vi "FPGA_initialize.vi"(2 "error in":errorcluster) -> (0 "error out":errorcluster)   [LabVIEW 2015]
uses:
  <vilib>/FPGAPlugInAG/PCIe-7841R/niLvFpga_Open_PCIe-7841R.vi
  <vilib>/rvi/interface/common/dynamic/niFpgaDynamicAddResources.vi
  <vilib>/FPGAPlugInAG/Dynamic/niLvFpga_Abort_Dynamic.vi
  <vilib>/FPGAPlugInAG/Dynamic/niLvFpga_Reset_Dynamic.vi
  <vilib>/FPGAPlugInAG/Dynamic/niLvFpga_Close_Dynamic.vi
  <vilib>/rvi/interface/nirviOpenFPGA/nirviOpenFPGA.xnode
  FPGA/FPGA Bitfiles/FPGAv0_FPGATarget_FPGAtriggercamer_zs8MuLZc0ko.lvbitx
  <vilib>/rvi/interface/nirviMethod/nirviMethod.xnode
  <vilib>/rvi/interface/nirviCloseFPGA/nirviCloseFPGA.xnode
  FPGA/FPGA Bitfiles/FPGAv0_FPGATarget_FPGAmeasureQPDsi_91djMVJ3FxY.lvbitx
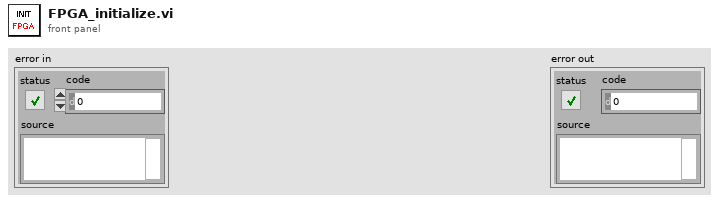
[diagram p1: front panel]
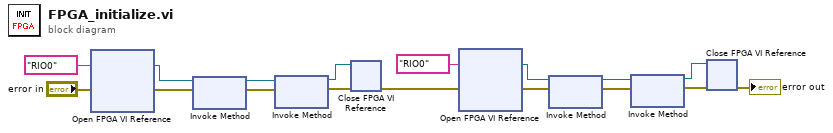
[diagram p0: block diagram]
diagram:
  n1 = xnode "Open FPGA VI Reference"("error in"="error in", "resource name"=tag "RIO0") -> ("FPGA VI Reference Out"=w14:refnum<k20>, "error out"=w15:errorcluster)
  n2 = xnode "Invoke Method"("FPGA VI Reference In"=w14, "error in"=w15) -> ("FPGA VI Reference Out"=w13:refnum<k20>, "error out"=w12:errorcluster)
  n3 = xnode "Invoke Method"("FPGA VI Reference In"=w13, "error in"=w12) -> ("FPGA VI Reference Out"=w10:refnum<k20>, "error out"=w11:errorcluster)
  n4 = xnode "Close FPGA VI Reference"("FPGA VI Reference In"=w10, "error in"=w11) -> ("error out"=w9:errorcluster)
  n5 = xnode "Open FPGA VI Reference"("error in"=w9, "resource name"=tag "RIO0") -> ("FPGA VI Reference Out"=w2:refnum<k20>, "error out"=w3:errorcluster)
  n6 = xnode "Invoke Method"("FPGA VI Reference In"=w2, "error in"=w3) -> ("FPGA VI Reference Out"=w4:refnum<k20>, "error out"=w5:errorcluster)
  n7 = xnode "Invoke Method"("FPGA VI Reference In"=w4, "error in"=w5) -> ("FPGA VI Reference Out"=w7:refnum<k20>, "error out"=w6:errorcluster)
  n8 = xnode "Close FPGA VI Reference"("FPGA VI Reference In"=w7, "error in"=w6) -> ("error out"=→"error out":errorcluster)
